vi "ADC.vi"() -> ()   [LabVIEW 2013]
uses:
  <vilib>/Platform/TimedLoop/XDataNode/timing_clust.ctl
  <vilib>/Platform/TimedLoop/XDataNode/nitl_modes.ctl
  <vilib>/Platform/TimedLoop/XDataNode/wakeup.ctl
  <vilib>/rvi/eio/common/nirviEmuTemplateMethod_errors.vi
  <vilib>/rvi/Emulation/niFpgaSctlEmulationGetInTimedLoop.vi
  <vilib>/rvi/Emulation/niFpgaEmulationReportErrorSimple.vi
  <vilib>/rvi/Emulation/niFpgaGetClockAttributes.vi
  <vilib>/rvi/Emulation/niFpgaCriticalErrorInLSC.vi
  <vilib>/platform/TimedLoop/XDataNode/XDataNode.xnode
  <vilib>/eio/EIONode/EIONode.xnode
  <vilib>/Platform/TimedLoop/XDataNode/XDNodeRunTimeDep.lvlib
panel:
  in  "48":u8=48
  in  "CDS1_1":u8=20
  in  "CDS1_2":u8=24
  in  "CDS2_1":u8=36
  in  "CDS2_2":u8=47
  in  "ADC_1":u8=20
  in  "ADC_2":u8=41
  in  "Стоп-цикл":bool
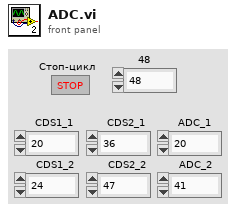
[diagram p1: front panel]
types:
  T1 = typedef "XDNodeRunTimeDep.lvlib/timing_clust.ctl" = cluster{"Expected End [f-1]":u64, "Actual End [f-1]":u64, "Finished Late? [f-1]":bool, "Expected End [i-1]":u64, "Actual End [i-1]":u64, "Finished Late? [i-1]":bool, "Expected Start [i]":u64, "Actual Start [i]":u64, "Expected Start [f]":u64, "Actual Start [f]":u64, "Source Name":string, "Structure Name":string, "Period":i64, "Deadline":i64, "Offset":i64, "Start":i64, "Priority":i32, "Timeout":i32, "Mode":T2, "Wakeup Reason":T3, "Error":errorcluster, "Source Type":string, "Secondary Source Type":string, "Global End Time":u64, "Global Start Time":u64, "Frame Duration":u64, "Iteration Duration":u64, "Assigned CPU":i32, "I/O Scan Engine Mode":u32}
  T2 = typedef "XDNodeRunTimeDep.lvlib/nitl_modes.ctl" = enum32{"No Change", "Process missed periods, maintain original phase", "Discard missed periods, maintain original phase", "Process missed periods, ignore original phase", "Discard missed periods, ignore original phase"}
  T3 = typedef "XDNodeRunTimeDep.lvlib/wakeup.ctl" = enum32{"Normal", "Aborted", "Asynchronous wakeup", "Timing source error", "Timed loop error", "Timeout"}
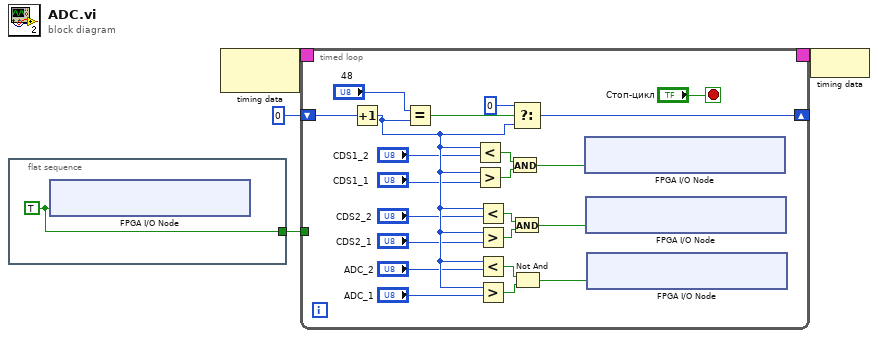
[diagram p0: block diagram]
diagram:
  n1 = flat-sequence {
    tunnel: [w5] -> w1
    frame #0 {
      w5 = TRUE ("IO Module\\DDCA_DIO0-7_WE")
      n2 = xnode "FPGA I/O Node"("IO Module\\DDCA_DIO0-7_WE"=w5) -> ()  [unwired: 1 in, 1 out]
    }
  }
  n3 = node-c288() -> (w4:T1)  [unwired: 1 in]
  n4 = timed-loop {
    timing: w4 -> [_]
    timing-out: [_] -> w3
    shift-right: [w16] -> _
    shift-left: u8 0 -> [w20]
    tunnel: w1 -> [_]
    stop <- "Стоп-цикл" stop-if-true
    n5 = Increment(x=w20) -> (x+1=w15:u8)
    n6 = Equal?(x="48", y=w15) -> (x = y?=w18:bool)
    n7 = Less?(x=w15, y="CDS1_2") -> (x < y?=w26:bool)
    n8 = Greater?(x=w15, y="CDS1_1") -> (0:w25:bool)
    n9 = Less?(x=w15, y="CDS2_2") -> (x < y?=w23:bool)
    n10 = Greater?(x=w15, y="CDS2_1") -> (0:w24:bool)
    n11 = Less?(x=w15, y="ADC_2") -> (x < y?=w22:bool)
    n12 = Greater?(x=w15, y="ADC_1") -> (0:w21:bool)
    n13 = And(x=w26, y=w25) -> (x .and. y?=w8:bool)
    n14 = Select(t=u8 0, s=w18, f=w15) -> (s? t:f=w16:u8)
    n15 = And(x=w23, y=w24) -> (x .and. y?=w7:bool)
    n16 = Not And(1:w21, 2:w22) -> (0:w6:bool)
    n17 = xnode "FPGA I/O Node"("IO Module\\DDCA_DIO0_Write"=w8) -> ()  [unwired: 1 in, 1 out]
    n18 = xnode "FPGA I/O Node"("IO Module\\DDCA_DIO1_Write"=w7) -> ()  [unwired: 1 in, 1 out]
    n19 = xnode "FPGA I/O Node"("IO Module\\DDCA_DIO2_Write"=w6) -> ()  [unwired: 1 in, 1 out]
  }
  n20 = node-c288(w3) -> ()
